vi "Test Get Code Coverage for Project Ignores Framework.vi"(8 "error in (no error)":errorcluster, 11 "Test Case In":refnum<class "Coverage Test.lvclass">) -> (0 "error out":errorcluster, 3 "Test Case Out":refnum<class "Coverage Test.lvclass">)   [LabVIEW 2020, in "LUnit Tests.lvlib" / "Coverage Test.lvclass"]
uses:
  Coverage Test.lvclass
  01074fa8-ee8a-411d-bc8b-fc92c4f90959.vi
  source/Framework/Coverage Analyzer/Coverage Analyzer.lvclass
  Test Dummys/Test Case Test Double/Test Case Test Double.lvclass
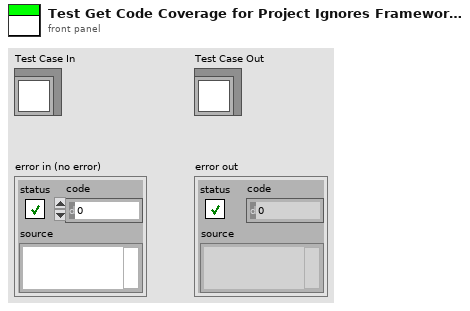
[diagram p1: front panel]
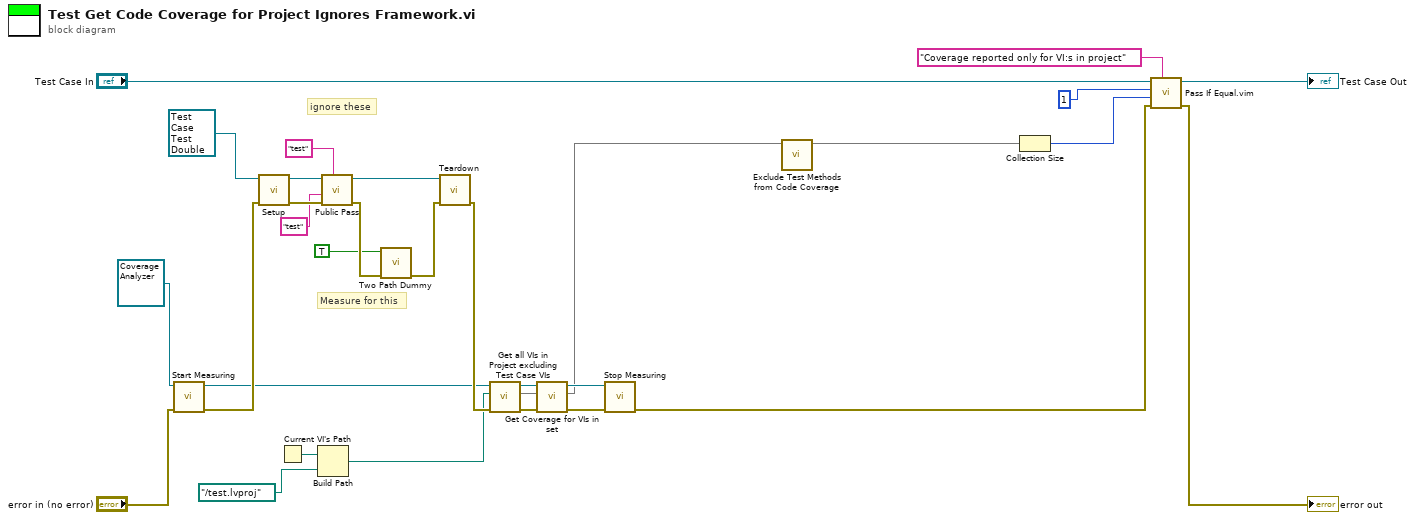
[diagram p0: block diagram]
diagram:
  # "ignore these"
  # "ignore these"
  # "ignore these"
  # "Measure for this"
  n1 = call "Start Measuring.vi"("error in (no error)"="error in (no error)", "Coverage Analyzer in"=refnum<class "Coverage Analyzer.lvclass"> refnum) -> ("error out"=w13:errorcluster, "Coverage Analyzer out"=w4:refnum<class "Coverage Analyzer.lvclass">)  [unwired: 8 in]
  n2 = call-dynamic "Setup.vi"("error in (no error)"=w13, "Test Case Test Double In"=refnum<class "Test Case Test Double.lvclass"> refnum ("Test Case Test Double in")) -> ("error out"=w18:errorcluster, "Test Case Test Double Out"=w15:refnum<class "Test Case Test Double.lvclass">)  [unwired: 8 in]
  n3 = Current VI's Path() -> (path=w10:path)
  n4 = Build Path(base path=w10, name or relative path=path "../test.lvproj") -> (appended path=w2:path)
  n5 = call "Public Pass.vi"("Description"="test", "error in (no error)"=w18, "Message"="test", "Test Case Test Double in"=w15) -> ("error out"=w8:errorcluster, "Test Case Test Double out"=w17:refnum<class "Test Case Test Double.lvclass">)  [unwired: 6 in]
  n6 = call "Two Path Dummy.vi"("error in (no error)"=w8, "Boolean"=TRUE) -> ("error out"=w7:errorcluster)  [unwired: 9 in]
  n7 = call-dynamic "Teardown.vi"("error in (no error)"=w7, "Test Case Test Double In"=w17) -> ("error out"=w14:errorcluster)  [unwired: 8 in, 1 out]
  n8 = call "Get all VIs in Project excluding Test Case VIs.vi"("error in (no error)"=w14, "Path"=w2, "Coverage Analyzer in"=w4) -> ("error out"=w5:errorcluster, "VIs"=w1:set{path}, "Coverage Analyzer out"=w3:refnum<class "Coverage Analyzer.lvclass">)  [unwired: 6 in]
  n9 = call "Get Coverage for VIs in set.vi"("error in (no error)"=w5, "VIs"=w1, "Coverage Analyzer in"=w3) -> ("error out"=w24:errorcluster, "Code Coverage"=w21:map{path, dbl}, "Coverage Analyzer out"=w23:refnum<class "Coverage Analyzer.lvclass">)  [unwired: 6 in]
  n10 = call "Stop Measuring.vi"("error in (no error)"=w24, "Coverage Analyzer in"=w23) -> ("error out"=w26:errorcluster)  [unwired: 8 in, 1 out]
  n11 = call "Exclude Test Methods from Code Coverage.vi"("Code Coverage"=w21) -> ("Filtered Code Coverage"=w20:map{path, dbl})  [unwired: 10 in]
  n12 = Collection Size(1:w20) -> (0:w19:i32)
  n13 = call "Pass If Equal.vim"("Description"="Coverage reported only for VI:s in project", "error in (no error)"=w26, "Actual"=w19, "Expected"=1 ("size"), "LUnit Test Case In"="Test Case In") -> ("error out"=→"error out":errorcluster, "LUnit Test Case Out"=→"Test Case Out":refnum<class "Coverage Test.lvclass">)  [unwired: 5 in]
